vi "Clear.vi"(7 "array in":T1) -> (3 "array out":T1)   [LabVIEW 2012, in "TLB` Template.lvlib" / "Tools_KeyedArray.lvlib"]
doc: "Returns an empty keyed array."
uses:
  Tools_KeyedArray.lvlib
  KeyedArray.ctl
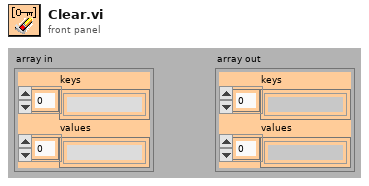
[diagram p1: front panel]
types:
  T1 = typedef "TLB` Template.lvlib/Tools_KeyedArray.lvlib/KeyedArray.ctl" = cluster{"keys":string[], "values":string[]}
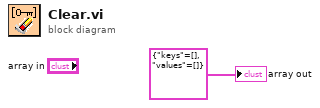
[diagram p0: block diagram]
diagram:
  "array out" <- T1 {"keys"=[], "values"=[]} ("array out")
